vi "Keithley 24XX Read Single.vi"() -> ()   [LabVIEW 2018]
doc: "This example shows how to configure a measurement and take a reading."
uses:
  Keithley 24XX.lvlib
  Public/Data/Read (Single Point).vi
panel:
  in  "Source Mode  (0: Voltage)":u16(ring) items=["Voltage", "Current"]
  in  "Compliance  Level (0.1)":dbl=0.1
  in  "Output Level (0)":dbl
  in  "Enable Resistance Auto Range (T:Enable)":bool=TRUE
  in  "Enable Current Auto Range (T:Enable)":bool=TRUE
  in  "Enable Voltage Auto Range (T:Enable)":bool=TRUE
  in  "Resistance Manual Range (1.0)":dbl=1.0
  in  "Current Manual Range (1.0)":dbl=1.0
  in  "Voltage Manual Range (1.0)":dbl=1.0
  out "Resistance":sgl
  out "Current":sgl
  out "Voltage":sgl
  in  "Serial Configuration":T1={"Baud Rate"=9600, "Parity"=0, "Data Bits"=8, "Stop Bits"=10, "Flow Control"=0} {"Flow Control" items=["None", "XON/XOFF", "RTS/CTS", "XON/XOFF & RTS/CTS", "DTR/DSR", "XON/XOFF & DTR/DSR"]; "Stop Bits" items=["1.0"=10, "1.5"=15, "2.0"=20]; "Data Bits" items=["7"=7, "8"=8]; "Parity" items=["None", "Odd", "Even", "Mark", "Space"]; "Baud Rate" items=["300"=300, "600"=600, "1200"=1200, "2400"=2400, "4800"=4800, "9600"=9600, "19200"=19200]}
  in  "VISA resource name":refnum<visa-resource-name>
  # "(c) 2006 National Instruments.  ALL RIGHTS RESERVED."
  # "(c) 2006 - 2015 National Instruments.  ALL RIGHTS RESERVED."
  # "Source Settings"
  # "Voltage Range Settings"
  # "Current Range Settings"
  # "Resistance Range Settings"
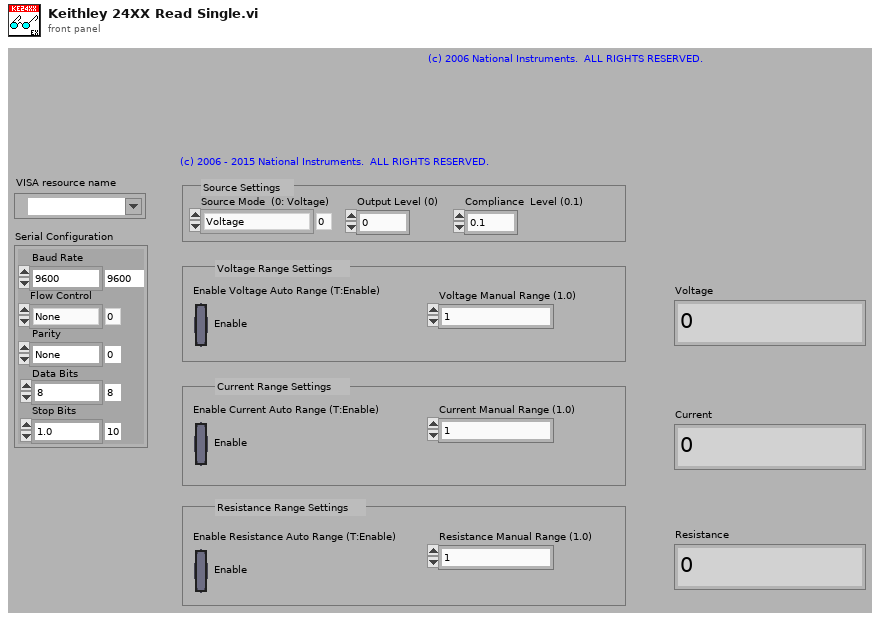
[diagram p1: front panel]
types:
  T1 = cluster{"Baud Rate":u32, "Parity":u16, "Data Bits":u16, "Stop Bits":u16, "Flow Control":u16}
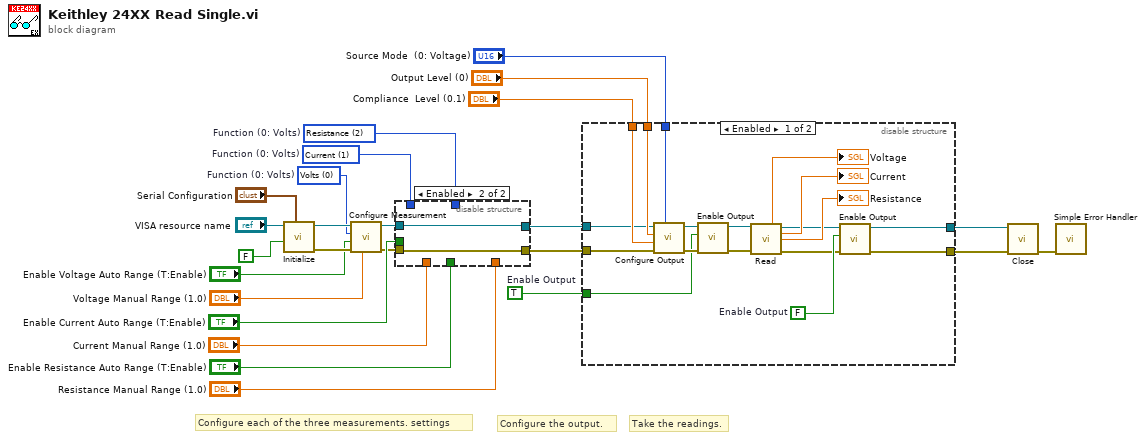
[diagram p0: block diagram]
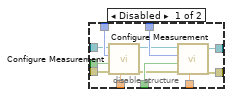
[diagram p2: hidden frame]
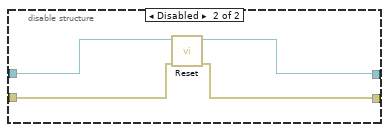
[diagram p3: hidden frame]
diagram:
  w7 = TRUE  # Enable Output
  w18 = u16 2 items=["Volts", "Current", "Resistance"]  # Function (0: Volts)
  w19 = u16 1 items=["Volts", "Current", "Resistance"]  # Function (0: Volts)
  w20 = u16 0 items=["Volts", "Current", "Resistance"]  # Function (0: Volts)
  # "Take the readings."
  # "Configure the output."
  # "Configure each of the three measurements. settings"
  n1 = call "Initialize.vi"("Serial Configuration"="Serial Configuration", "Reset (True)"=FALSE, "VISA resource name"="VISA resource name") -> ("error out"=w21:errorcluster, "VISA resource name out"=w22:refnum<visa-resource-name>)  [unwired: 7 in]
  n2 = call "Configure Measurement.vi"("Manual Range (1.0)"="Voltage Manual Range (1.0)", "error in (no error)"=w21, "Enable Auto Range (T:Enable)"="Enable Voltage Auto Range (T:Enable)", "Function (0: Volts)"=w20, "VISA resource name"=w22) -> ("error out"=w1:errorcluster, "VISA resource name out"=w2:refnum<visa-resource-name>)  [unwired: 5 in]
  n3 = disable-structure shown="Enabled" {
    disable-tunnel: w19 -> [w37 _]
    disable-tunnel: w18 -> [w36 _]
    disable-tunnel: "Current Manual Range (1.0)" -> [w35 _]
    disable-tunnel: "Resistance Manual Range (1.0)" -> [w34 _]
    disable-tunnel: "Enable Current Auto Range (T:Enable)" -> [w33 _]
    disable-tunnel: "Enable Resistance Auto Range (T:Enable)" -> [w32 _]
    disable-tunnel: [w31 w38] -> w6
    disable-tunnel: [w30 w39] -> w5
    disable-tunnel: w2 -> [w29 w39]
    disable-tunnel: w1 -> [w28 w38]
    frame Disabled {
      n4 = call "Configure Measurement.vi"("Manual Range (1.0)"=w35, "error in (no error)"=w28, "Enable Auto Range (T:Enable)"=w33, "Function (0: Volts)"=w37, "VISA resource name"=w29) -> ("error out"=w27:errorcluster, "VISA resource name out"=w26:refnum<visa-resource-name>)  [unwired: 5 in]
      n5 = call "Configure Measurement.vi"("Manual Range (1.0)"=w34, "error in (no error)"=w27, "Enable Auto Range (T:Enable)"=w32, "Function (0: Volts)"=w36, "VISA resource name"=w26) -> ("error out"=w31:errorcluster, "VISA resource name out"=w30:refnum<visa-resource-name>)  [unwired: 5 in]
    }
    frame Enabled {
    }
  }
  n6 = disable-structure shown="Enabled" {
    disable-tunnel: "Output Level (0)" -> [w53 _]
    disable-tunnel: "Compliance  Level (0.1)" -> [w52 _]
    disable-tunnel: [w51 w60] -> w9
    disable-tunnel: [w50 w58] -> w8
    disable-tunnel: w7 -> [w43 _]
    disable-tunnel: w6 -> [w42 w59]
    disable-tunnel: w5 -> [w41 w61]
    disable-tunnel: "Source Mode  (0: Voltage)" -> [w40 _]
    frame Enabled {
      w54 = FALSE  # Enable Output
      n7 = call "Configure Output.vi"("Source Mode  (0: Voltage)"=w40, "error in (no error)"=w42, "Compliance  Level (0.1)"=w52, "Output Level (0)"=w53, "VISA resource name"=w41) -> ("error out"=w44:errorcluster, "VISA resource name out"=w45:refnum<visa-resource-name>)  [unwired: 5 in]
      n8 = call "Enable Output.vi"("error in (no error)"=w44, "Enable Output (T: Enable)"=w43, "VISA resource name"=w45) -> ("error out"=w47:errorcluster, "VISA resource name out"=w46:refnum<visa-resource-name>)  [unwired: 7 in]
      n9 = call-poly "Read.vi"("VISA resource name"=w46, "error in (no error)"=w47) -> ("Voltage"=→"Voltage":sgl, "VISA resource name out"=w48:refnum<visa-resource-name>, "Current"=→"Current":sgl, "Resistance"=→"Resistance":sgl, "error out"=w49:errorcluster)  [unwired: 7 in, 2 out]
      n10 = call "Enable Output.vi"("error in (no error)"=w49, "Enable Output (T: Enable)"=w54, "VISA resource name"=w48) -> ("error out"=w50:errorcluster, "VISA resource name out"=w51:refnum<visa-resource-name>)  [unwired: 7 in]
    }
    frame Disabled {
      n11 = call "Reset.vi"("error in (no error)"=w59, "VISA resource name"=w61) -> ("error out"=w58:errorcluster, "VISA resource name out"=w60:refnum<visa-resource-name>)  [unwired: 8 in]
    }
  }
  n12 = call "Close.vi"("error in (no error)"=w8, "VISA resource name"=w9) -> ("error out"=w25:errorcluster)  [unwired: 9 in]
  n13 = call <vilib>:"Simple Error Handler.vi"("error in (no error)"=w25) -> ()  [unwired: 4 in, 5 out]
